vi "ConvertTo(SGL).vi"(8 "error in":errorcluster, 9 "Message Payload":variant) -> (0 "error out":errorcluster, 1 "Message Payload SGL Numeric":sgl)   [LabVIEW 2017]
doc: "Convert variant to SGL scalar\n\nBolder Software LLC"
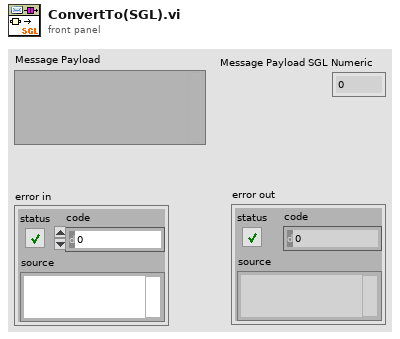
[diagram p1: front panel]
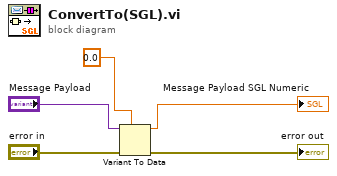
[diagram p0: block diagram]
diagram:
  n1 = Variant To Data(error in="error in", type=sgl 0.0 ("Message Payload DBL Numeric"), Variant="Message Payload") -> (data=→"Message Payload SGL Numeric":sgl, error out=→"error out":errorcluster)
